vi "TEMPERATURE PROJECTALL LEDl  run.vi"() -> ()   [LabVIEW 2019]
panel:
  in  "stop (T) 5":bool=TRUE caption="stop (T)"
  in  "stop (T) 4":bool=TRUE caption="stop (T)"
  in  "stop (T) 3":bool=TRUE caption="stop (T)"
  out "MODERATE":bool
  out "Meter":dbl(knob) scale=-2.5..2.5
  in  "stop (T)":bool=TRUE
  in  "STOP":bool
  out "Waveform Chart":dynamicdata(graph)
  out "TANK":dbl(slide) scale=-2.5..2.5
  out "TEMPERATURE":dbl
  out "LOW":bool
  out "HIGH":bool
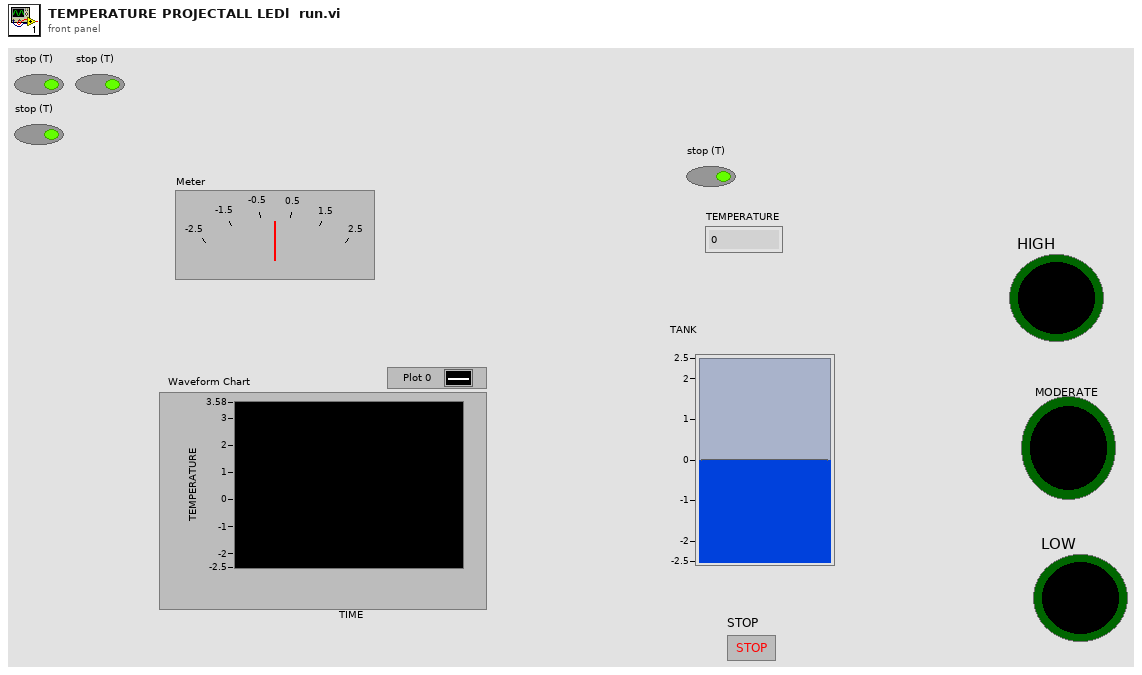
[diagram p1: front panel]
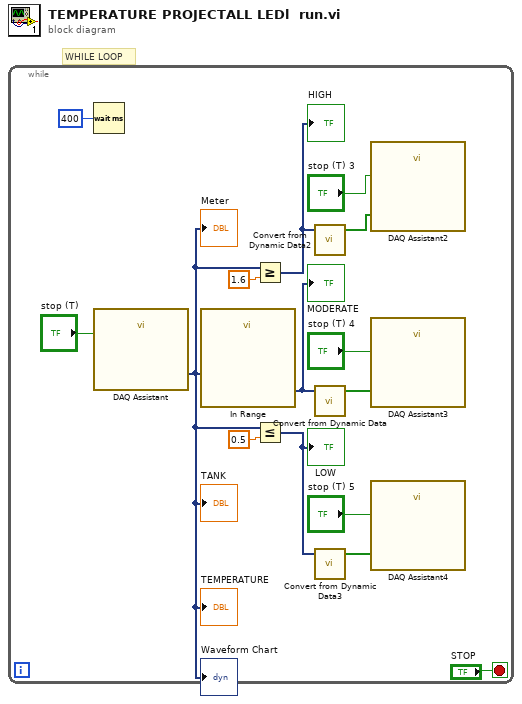
[diagram p0: block diagram]
diagram:
  # "WHILE LOOP"
  n1 = while {
    stop <- "STOP" stop-if-true
    n2 = Wait (ms)(milliseconds to wait=u32 400) -> ()  [unwired: 1 out]
    n3 = call "DAQ Assistant"("stop (T)"="stop (T)") -> ("data"=w6:dynamicdata)  [unwired: 16 in, 2 out]
    "TEMPERATURE" <- w6
    "TANK" <- w6
    "Waveform Chart" <- w6
    "Meter" <- w6
    n4 = call "In Range"("Operand 1"=w6) -> ("Result"=w10:dynamicdata)  [unwired: 9 in, 1 out]
    "MODERATE" <- w10
    n5 = Greater Or Equal?(x=w6, y=1.6) -> (x >= y?=w8:dynamicdata)
    "HIGH" <- w8
    n6 = Less Or Equal?(x=w6, y=0.5) -> (x <= y?=w5:dynamicdata)
    "LOW" <- w5
    n7 = call "Convert from Dynamic Data2"("Dynamic Data Type"=w8) -> ("Array"=w7:bool[])  [unwired: 3 in]
    n8 = call "Convert from Dynamic Data"("Dynamic Data Type"=w10) -> ("Array"=w9:bool[])  [unwired: 3 in]
    n9 = call "Convert from Dynamic Data3"("Dynamic Data Type"=w5) -> ("Array"=w4:bool[])  [unwired: 3 in]
    n10 = call "DAQ Assistant2"("data"=w7, "stop (T)"="stop (T) 3") -> ()  [unwired: 16 in, 2 out]
    n11 = call "DAQ Assistant3"("data"=w9, "stop (T)"="stop (T) 4") -> ()  [unwired: 16 in, 2 out]
    n12 = call "DAQ Assistant4"("data"=w4, "stop (T)"="stop (T) 5") -> ()  [unwired: 16 in, 2 out]
  }
